vi "Enable Message Logging.vi"(8 "error in (no error)":errorcluster, 11 "Monitored Actor in":refnum<class "Monitored Actor.lvclass">) -> (0 "error out":errorcluster, 3 "Monitored Actor out":refnum<class "Monitored Actor.lvclass">)   [LabVIEW 2023, in "Monitored Actor.lvlib" / "Monitored Actor.lvclass"]
doc: "Starts reporting all messages received to the message logger\n\nCopyright: MGI 2016\nAuthor: Derek Trepanier"
uses:
  Monitored Actor.lvclass
  Monitored Actor.lvclass/Monitored Actor.ctl
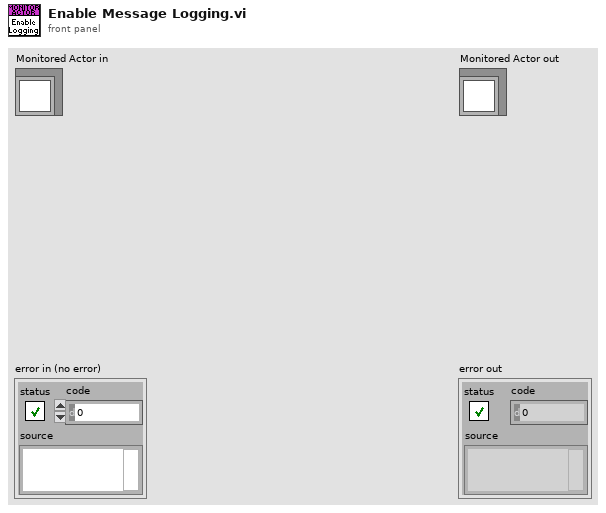
[diagram p1: front panel]
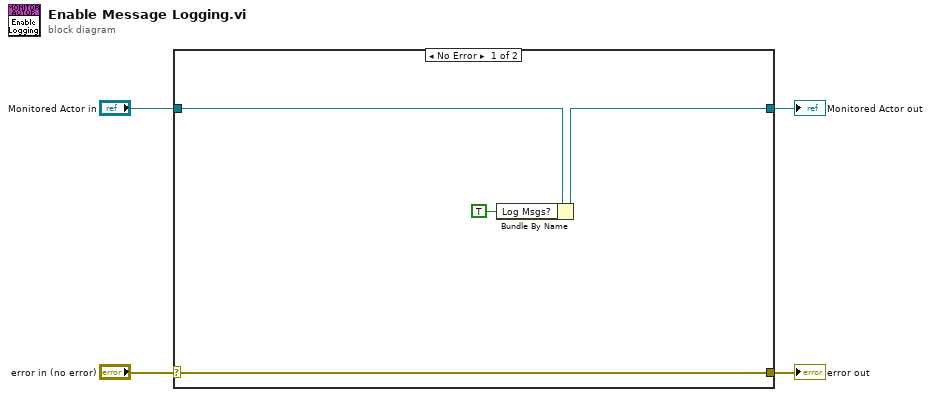
[diagram p0: block diagram]
diagram:
  n1 = case shown="No Error" "error in (no error)" {
    selector: "error in (no error)" -> [w6 w10]
    tunnel: [w6 w10] -> w3
    tunnel: [w7 w9] -> w1
    tunnel: "Monitored Actor in" -> [w8 w9]
    frame No Error {
      n2 = Bundle By Name(cluster=w8, "Log Msgs?"=TRUE) -> (w7:refnum<class "Monitored Actor.lvclass">)
    }
    frame Error {
    }
  }
  "error out" <- w3
  "Monitored Actor out" <- w1
